vi "Test_Cache.vi"() -> ()   [LabVIEW 2016, in "Motor Base.lvlib"]
uses:
  Motor Base.lvlib
panel:
  out "x*y":dbl
  out "Transmit PDO mapping 4-Position actual value":i32
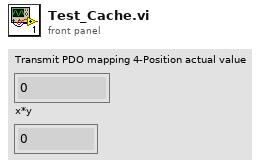
[diagram p1: front panel]
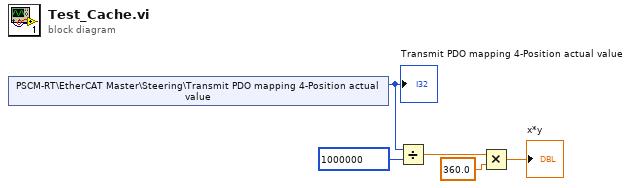
[diagram p0: block diagram]
diagram:
  n1 = shared-variable "PSCM-RT\\EtherCAT Master\\Steering\\Transmit PDO mapping 4-Position actual value"() -> (w5:i32)  [unwired: 1 in, 1 out]
  "Transmit PDO mapping 4-Position actual value" <- w5
  n2 = Divide(x=w5, y=1000000) -> (x/y=w3:dbl)
  n3 = Multiply(x=w3, y=360.0) -> (x*y=→"x*y":dbl)
